vi "Configure Run UTF.vi"(8 "error in (no error)":errorcluster, 11 "JSON string":string) -> (0 "error out":errorcluster, 3 "Run UTF.lvclass":refnum<class "Run UTF.lvclass">)   [LabVIEW 2014, in "Run UTF.lvclass"]
uses:
  Run UTF.lvclass
  Run UTF - STYP.ctl
  Run UTF.lvclass/Run UTF.ctl
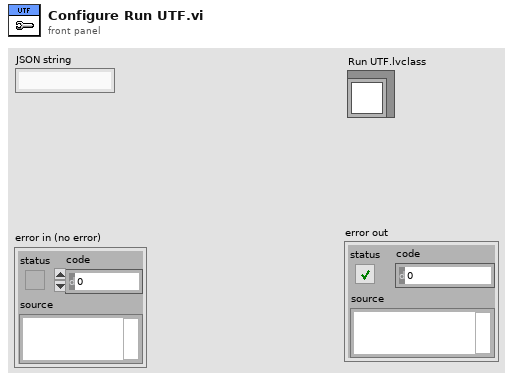
[diagram p1: front panel]
types:
  T1 = typedef "Run UTF - STYP.ctl" = cluster{"Project Path":string}
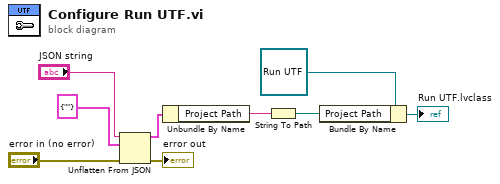
[diagram p0: block diagram]
diagram:
  n1 = Unflatten From JSON(JSON string="JSON string", type and defaults=T1 {"Project Path"=""} ("Run UTF"), error in (no error)="error in (no error)") -> (value=w6:T1, error out=→"error out":errorcluster)  [unwired: 4 in]
  n2 = Unbundle By Name(w6) -> ("Project Path"=w5:string)
  n3 = String To Path(string=w5) -> (path=w4:path)
  n4 = Bundle By Name(cluster=refnum<class "Run UTF.lvclass"> refnum ("Run UTF.lvclass"), "Project Path"=w4) -> (→"Run UTF.lvclass":refnum<class "Run UTF.lvclass">)
